vi "Globals - RT Stream.vi"() -> ()   [LabVIEW 2017]
uses:
  Support/Message Queue/Message Cluster.ctl
  Support/Message Queue/Message Queue.lvlib
panel:
  in  "RT Writer Stream":refnum<k21>
  in  "UI Reader Stream":refnum<k21>
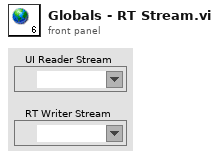
[diagram p1: front panel]
diagram:
